vi "Insert Bus Monitor.vi"(8 "error in (no error)":errorcluster, 10 "Protected Subpanel":T1, 11 "IMediator In":refnum<class "IMediator.lvclass">) -> (0 "error out":errorcluster, 3 "IMediator Out":refnum<class "IMediator.lvclass">)   [LabVIEW 2017, in "IMediator.lvlib" / "IMediator.lvclass"]
uses:
  IMediator.lvclass
  IViewable/ProtectedSubpanel/Protected Subpanel Reference.ctl
  IViewable/ProtectedSubpanel/ProtectedSubpanel.lvclass
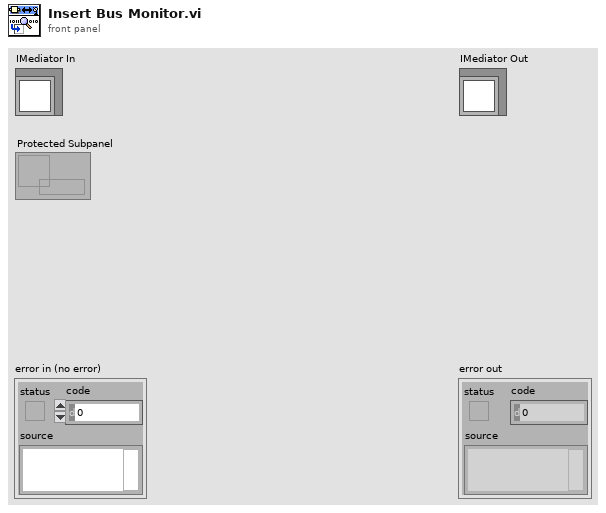
[diagram p1: front panel]
types:
  T1 = typedef "IViewable.lvlib/ProtectedSubpanel.lvclass/Protected Subpanel Reference.ctl" = refnum<data-value>
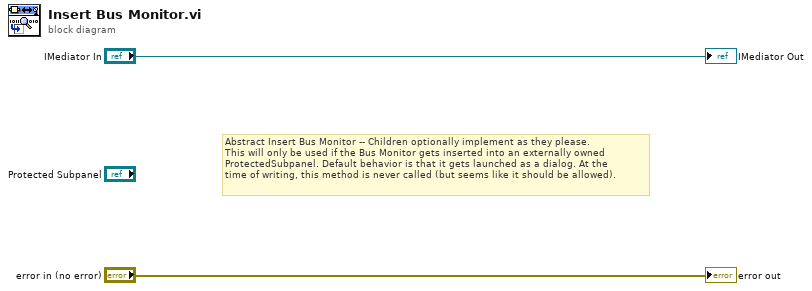
[diagram p0: block diagram]
diagram:
  # "Abstract Insert Bus Monitor -- Children optionally implement as they please.\nThis will only be used if the Bus Monitor gets inserted into an externally owned\nProtectedSubpanel. Default behavior is that it gets launched as a dialog. At the\ntime of writing, this method is never called (but seems like it should be allowed)."
  "error out" <- "error in (no error)"
  "IMediator Out" <- "IMediator In"
